vi "Space Reroute.vi"(9 "Deform Array":dbl[](array[numeric])=[1.0, 1.0, 1.0, 0.0, 0.0, 0.0, 0.0, 0.0, 0.0], 10 "Pivot Pt":dbl[](array[numeric])=[0.0, 5.0, 0.0], 11 "Nominal Traj Pt":dbl[](array[numeric])=[0.0, 10.0, 0.0]) -> (3 "Reroute Traj Pt":dbl[](array[numeric]))   [LabVIEW 2016]
doc: "This VI takes in input (x,y) coordinate, compensates for the EyeCenter offset, and output a deformed (x\",y\") using the following formula:\n\n[x',y']' = [x,y]' - EyeCenter;\n[x\",y\"]' = R(theta_z) * diag(x_scaling,y+scaling) * [x',y']' +[x_offset,y_offset]."
uses:
  <vilib>/Analysis/baseanly.llb/A x Vector.vi
  <vilib>/Analysis/Matrix/Numeric/Conversions/Array To Matrix - RA2.vi
  <vilib>/Analysis/NI_AALBase.lvlib
  <vilib>/Analysis/Matrix/NI_Matrix.lvlib
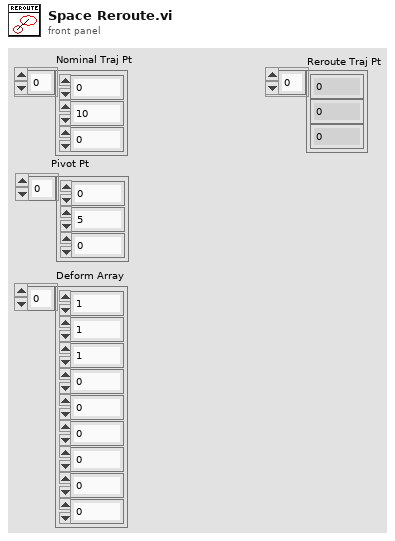
[diagram p1: front panel]
types:
  T1 = typedef "NI_Matrix.lvlib/RealMatrix.ctl" = dbl[][]
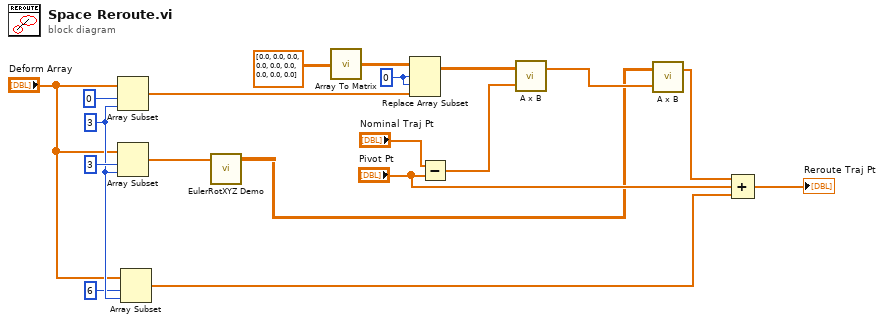
[diagram p0: block diagram]
diagram:
  w9 = 3 ("length")
  w17 = 0 ("disabled index (row)")
  n1 = Array Subset(array="Deform Array", index=0, length=w9) -> (w14:dbl[])
  n2 = Array Subset(array="Deform Array", index=3, length=w9) -> (w2:dbl[])
  n3 = Array Subset(array="Deform Array", index=6, length=w9) -> (w4:dbl[])
  n4 = call "EulerRotXYZ Demo.vi"("Euler Angle (XYZ)"=w2) -> ("Rotation Mtx"=w1:T1)  [unwired: 10 in]
  n5 = call-poly <vilib>:"Array To Matrix.vi"("Real 2D Array"=dbl[][] [[0.0, 0.0, 0.0], [0.0, 0.0, 0.0], [0.0, 0.0, 0.0]]) -> ("Real Matrix"=w18:T1)
  n6 = Replace Array Subset(array=w18, new element=w14, index (row)=w17, index (col)=w17) -> (w13:T1)
  n7 = Subtract(x="Nominal Traj Pt", y="Pivot Pt") -> (x-y=w12:dbl[])
  n8 = call-poly <vilib>:"A x B.vi"("Vector"=w12, "A"=w13) -> ("A x Vector"=w11:dbl[])  [unwired: 1 out]
  n9 = call-poly <vilib>:"A x B.vi"("Vector"=w11, "A"=w1) -> ("A x Vector"=w6:dbl[])  [unwired: 1 out]
  n10 = Compound Arithmetic op=ADD(w6, "Pivot Pt", w4) -> (→"Reroute Traj Pt":dbl[])
